vi "Read Instance Name.vi"(8 "error in (no error)":errorcluster, 11 "System Actor in":refnum<class "System Actor.lvclass">) -> (0 "error out":errorcluster, 2 "Instance Name":string, 3 "System Actor out":refnum<class "System Actor.lvclass">)   [LabVIEW 2014, in "Robot Actor Framework.lvlib" / "System Actor.lvlib" / "System Actor.lvclass"]
uses:
  System Actor.lvclass
  <vilib>/Utility/config.llb/Config Data RefNum.ctl
  System Actor.lvclass/System Actor.ctl
  <vilib>/Utility/config.llb/NI_LVConfig.lvlib
panel:
  out "refnum":T1
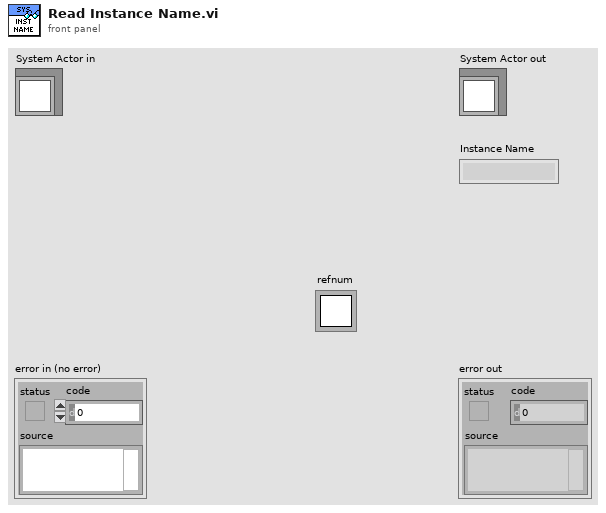
[diagram p1: front panel]
types:
  T1 = typedef "NI_LVConfig.lvlib/Config Data RefNum.ctl" = refnum<k1>
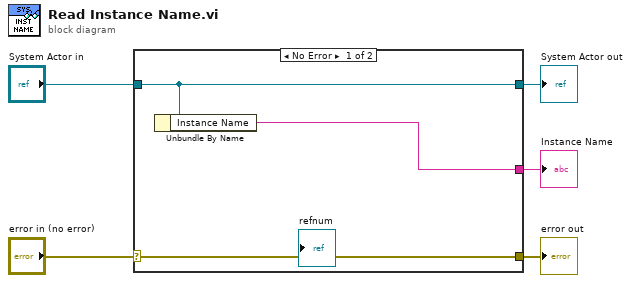
[diagram p0: block diagram]
diagram:
  n1 = case shown="No Error" "error in (no error)" {
    selector: "error in (no error)" -> [w8 w9]
    tunnel: [w8 w9] -> w4
    tunnel: [w7 w10] -> w2
    tunnel: "System Actor in" -> [w7 w10]
    tunnel: [w6 _] -> w1
    frame No Error {
      n2 = Unbundle By Name(w7) -> ("Instance Name"=w6:string)
    }
    frame Error {
    }
  }
  "error out" <- w4
  "System Actor out" <- w2
  "Instance Name" <- w1
